vi "LowPassFilter.vi"() -> ()   [LabVIEW 2017]
uses:
  <vilib>/express/express analysis/Spectral/Block/exnSpectralBlock spectral measurements RMS poly.vi
  <vilib>/express/express analysis/Spectral/Block/exnSpectralBlock spectral measurements RMS DDT.vi
  <vilib>/express/express analysis/Spectral/XNode/ExpressSpectralMeasurementsBlockNode.xnode
panel:
  out "Square":dynamicdata(graph)
  out "Waveform Graph 2":dynamicdata(graph)
  in  "stop":bool
  out "Waveform Graph":dynamicdata(graph)
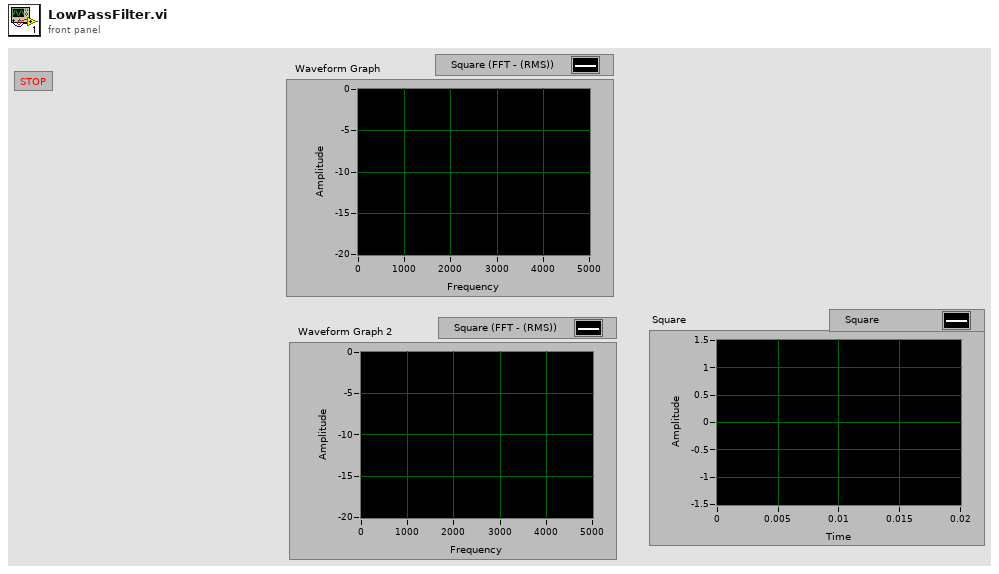
[diagram p1: front panel]
types:
  T1 = cluster{"averaging mode":u16, "weighting mode":u16, "number of averages":u32}
  T2 = cluster{"dB On (F)":bool, "unwrap phase (F)":bool, "convert to degree (F)":bool}
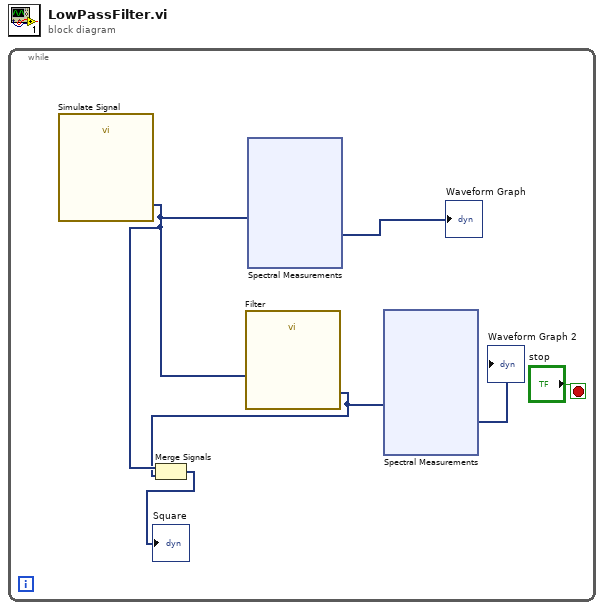
[diagram p0: block diagram]
diagram:
  n1 = while {
    stop <- "stop" stop-if-true
    n2 = call "Simulate Signal"() -> ("Square"=w4:dynamicdata)  [unwired: 14 in, 1 out]
    n3 = call "Filter"("Signal"=w4) -> ("Filtered Signal"=w1:dynamicdata)  [unwired: 9 in, 1 out]
    n4 = Merge Signals(w4, w1) -> (→"Square":dynamicdata)
    n5 = xnode "Spectral Measurements"("Signals"=w4) -> ("FFT - (RMS)"=→"Waveform Graph":dynamicdata)  [unwired: 1 in, 2 out]
    n6 = xnode "Spectral Measurements"("Signals"=w1) -> ("FFT - (RMS)"=→"Waveform Graph 2":dynamicdata)  [unwired: 1 in, 2 out]
  }
